vi "Open.vi"(8 "error in (no error)":errorcluster caption="entrée d'erreur (pas d'erreur)", 11 "Class Relay_Board usb_relay_device en entrée":refnum<class "Class Relay_Board usb_Relay_device.lvclass">) -> (0 "error out":errorcluster caption="sortie d'erreur", 3 "Class Relay_Board usb_relay_device en sortie":refnum<class "Class Relay_Board usb_Relay_device.lvclass">)   [LabVIEW 2020, in "Library Instrument & Equipement.lvlib" / "Library Relay_Board.lvlib" / "Class Relay_Board usb_Relay_device.lvclass"]
uses:
  Class Relay_Board usb_Relay_device.lvclass
  C:/Users/ngarcin/OneDrive - Altyor/Standard TB/Class/Relay_Board/Relay_Board (Default)/Class Relay_Board (Default).lvclass
  Class Relay_Board usb_Relay_device.lvclass/Class Relay_Board usb_Relay_device.ctl
  usb_relay_device/usb_relay_device.lvlib
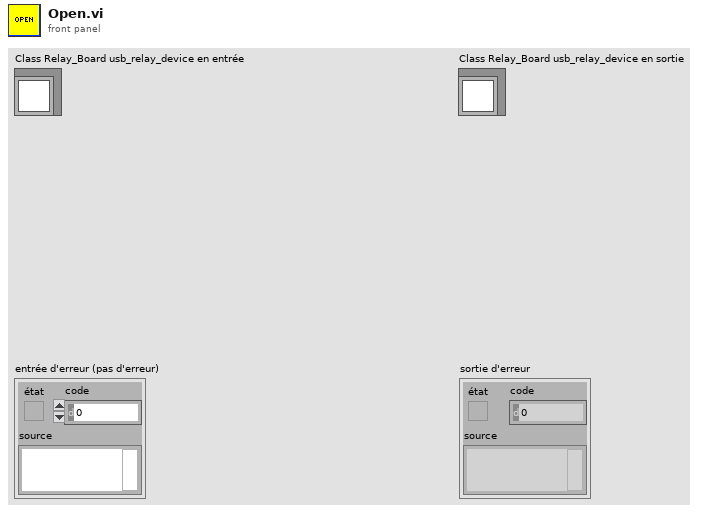
[diagram p1: front panel]
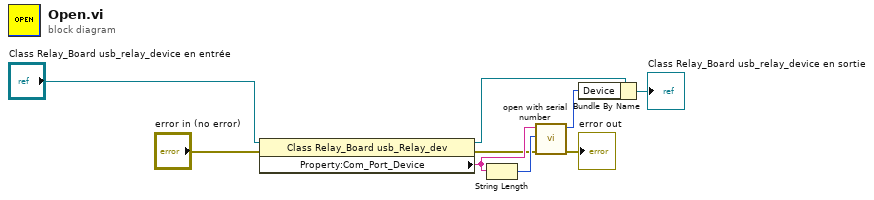
[diagram p0: block diagram]
diagram:
  n1 = property class="Class Relay_Board usb_Relay_dev"(reference="Class Relay_Board usb_relay_device en entrée", error in="error in (no error)") -> (reference out=w7:refnum<class "Class Relay_Board usb_Relay_device.lvclass">, error out=w3:errorcluster, "Property:Com_Port_Device"=w4:string)
  n2 = String Length(string=w4) -> (length=w5:i32)
  n3 = call "open with serial number.vi"("error in (no error)"=w3, "len"=w5, "serial_number"=w4) -> ("error out"=→"error out":errorcluster, "Handle"=w1:i32)  [unwired: 7 in]
  n4 = Bundle By Name(cluster=w7, "Device"=w1) -> (→"Class Relay_Board usb_relay_device en sortie":refnum<class "Class Relay_Board usb_Relay_device.lvclass">)
